vi "ROS_requestTopic.vi"(2 "Topic":string, 3 "Caller ID":string) -> (1 "XML":string)   [LabVIEW 2010]
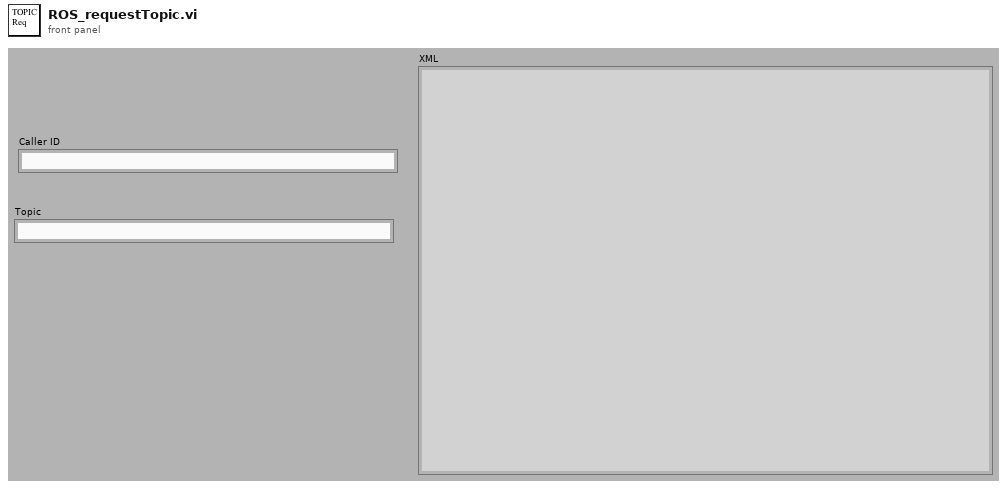
[diagram p1: front panel]
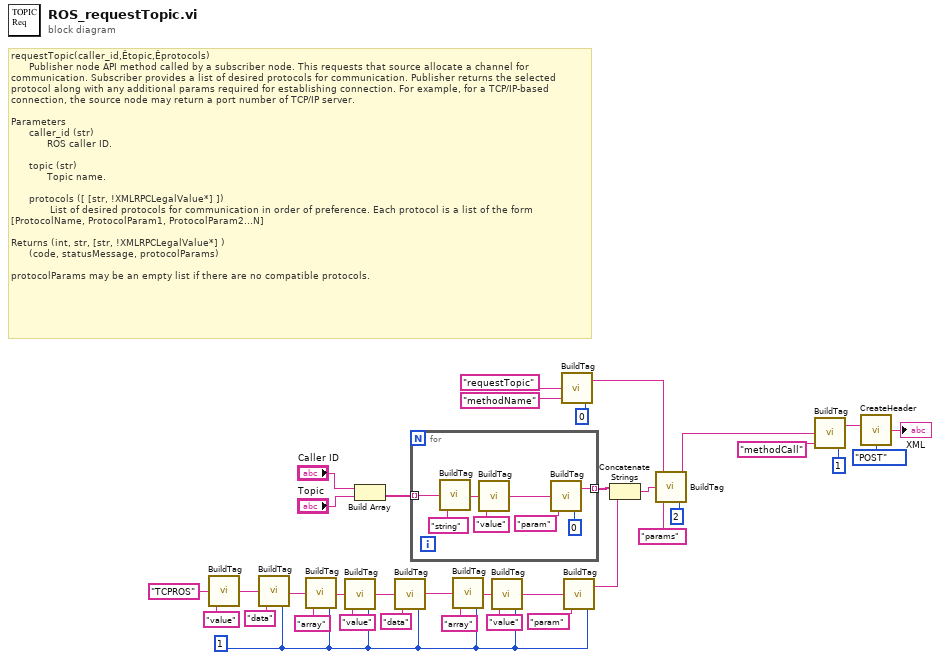
[diagram p0: block diagram]
diagram:
  w4 = i8 1 ("Indent")
  # "requestTopic(caller_id,Êtopic,Êprotocols)\n      Publisher node API method called by a subscriber node. This requests that source allocate a channel for communication. Subscriber provides a list of desired protocols for communication. Publisher returns the selected protocol along with any additional params required for establishing connection. For example, for a TCP/IP-based connection, the source node may return a port number of TCP/IP server. \n\nParameters \n      caller_id (str) \n            ROS caller ID.\n\n      topic (str) \n            Topic name.\n\n      protocols ([ [str, !XMLRPCLegalValue*] ]) \n             List of desired protocols for communication in order of preference. Each protocol is a list of the form [ProtocolName, ProtocolParam1, ProtocolParam2...N]\n\nReturns (int, str, [str, !XMLRPCLegalValue*] ) \n      (code, statusMessage, protocolParams) \n\nprotocolParams may be an empty list if there are no compatible protocols."
  n1 = call "BuildTag.vi"("tag"="value", "value"="TCPROS") -> ("string out"=w14:string)  [unwired: 2 in]
  n2 = call "BuildTag.vi"("Indent"=w4, "tag"="data", "value"=w14) -> ("string out"=w11:string)  [unwired: 1 in]
  n3 = call "BuildTag.vi"("Indent"=w4, "tag"="array", "value"=w11) -> ("string out"=w18:string)  [unwired: 1 in]
  n4 = call "BuildTag.vi"("Indent"=w4, "tag"="value", "value"=w18) -> ("string out"=w16:string)  [unwired: 1 in]
  n5 = Build Array("Caller ID", "Topic") -> (w1:string[])
  n6 = call "BuildTag.vi"("Indent"=w4, "tag"="data", "value"=w16) -> ("string out"=w15:string)  [unwired: 1 in]
  n7 = for {
    tunnel: w1 -> [w37] mode=indexing
    tunnel: [w36] -> w27 mode=indexing
    n8 = call "BuildTag.vi"("tag"="string", "value"=w37) -> ("string out"=w41:string)  [unwired: 2 in]
    n9 = call "BuildTag.vi"("tag"="value", "value"=w41) -> ("string out"=w39:string)  [unwired: 2 in]
    n10 = call "BuildTag.vi"("Indent"=i8 0, "tag"="param", "value"=w39) -> ("string out"=w36:string)  [unwired: 1 in]
  }
  n11 = call "BuildTag.vi"("Indent"=w4, "tag"="array", "value"=w15) -> ("string out"=w23:string)  [unwired: 1 in]
  n12 = call "BuildTag.vi"("Indent"=w4, "tag"="value", "value"=w23) -> ("string out"=w25:string)  [unwired: 1 in]
  n13 = call "BuildTag.vi"("Indent"=i8 0, "tag"="methodName", "value"="requestTopic" ("Method Name")) -> ("string out"=w30:string)  [unwired: 1 in]
  n14 = call "BuildTag.vi"("Indent"=w4, "tag"="param", "value"=w25) -> ("string out"=w9:string)  [unwired: 1 in]
  n15 = Concatenate Strings(w27, w9) -> (w26:string)
  n16 = call "BuildTag.vi"("Indent"=i8 2, "tag"="params", "value"=w26, "string in"=w30) -> ("string out"=w33:string)
  n17 = call "BuildTag.vi"("Indent"=i8 1, "tag"="methodCall", "value"=w33) -> ("string out"=w8:string)  [unwired: 1 in]
  n18 = call "CreateHeader.vi"("Content"=w8, "type"=enum16{"POST", "Reply"}."POST") -> ("XML"=→"XML":string)
